vi "MasterRobotModeController.vi"() -> (1 "FMS Robot Mode":T1, 2 "Auto Reset":bool, 3 "Robot is Autonomous":bool)   [LabVIEW 2019]
doc: "This state controller manages the Robot Mode and whether or not the robot is running autonomously. The robot will continue running autonomously after Autonomous Mode ends, until the driver touches the joystick during TeleOperated Mode or until/unless the FORCE HUMAN CONTROL override is flipped on the FRC 4265 Dashboard."
uses:
  <vilib>/Rock Robotics/WPI/DriverStation/WPI_DriverStationRobotMode2.ctl
  refnums.vi
  GRNF_Joystick.vi
  dsdata.vi
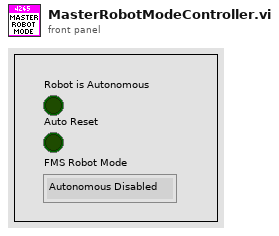
[diagram p1: front panel]
types:
  T1 = typedef "WPI_DriverStationRobotMode2.ctl" = enum16{"Autonomous Disabled", "Autonomous Enabled", "Teleop Disabled", "Teleop Enabled", "Disconnected", "Finish", "Test Disabled", "Test Enabled", "Emergency Stopped"}
  T2 = typedef "WPI_JoystickDevRef.ctl" = cluster{"Device":T3}
  T3 = typedef "WPI_JoystickDeviceEnum.ctl" = enum16{"USB 0", "USB 1", "USB 2", "USB 3", "USB 4", "USB 5"}
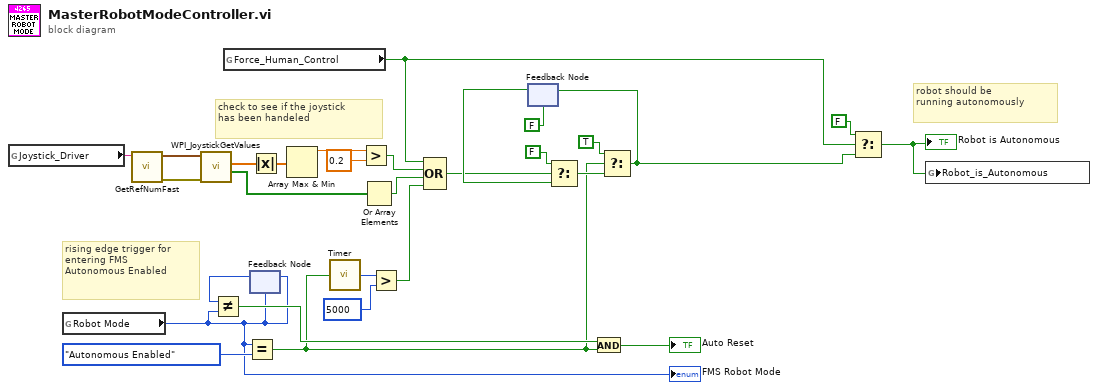
[diagram p0: block diagram]
diagram:
  # "rising edge trigger for\nentering FMS\nAutonomous Enabled"
  # "robot should be\nrunning autonomously"
  # "check to see if the joystick \nhas been handeled"
  n1 = global read "refnums.vi" "Joystick_Driver"() -> (w27:string)
  n2 = global read "dsdata.vi" "Robot Mode"() -> (w9:T1)
  "FMS Robot Mode" <- w9
  n3 = call-poly "GetRefNumFast.vi"("RefNum Name"=w27) -> ("Error"=w28:errorcluster, "Device Reference"=w29:T2)  [unwired: 5 in]
  n4 = call <vilib>:"WPI_JoystickGetValues.vi"("error in (no error)"=w28, "JoystickDevRef"=w29) -> ("Buttons"=w26:bool[], "Axes"=w25:dbl[])  [unwired: 5 in, 3 out]
  n5 = global read "dsdata.vi" "Force_Human_Control"() -> (w5:bool)
  n6 = Equal?(x=w9, y=WPI_DriverStationRobotMode2."Autonomous Enabled" ("Robot Mode")) -> (x = y?=w4:bool)
  n7 = feedback #1(w9) -> (w16:T1)
  n8 = Not Equal?(x=w16, y=w9) -> (x != y?=w15:bool)
  n9 = feedback-in #1(w9) -> ()
  n10 = Absolute Value(x=w25) -> (abs(x)=w24:dbl[])
  n11 = Array Max & Min(array=w24) -> (max value=w23:dbl)  [unwired: 3 out]
  n12 = call "Timer.vi"("Reset Timer"=w4) -> ("Time (ms)"=w3:u32)
  n13 = Greater?(x=w23, y=0.2) -> (0:w21:bool)
  n14 = Or Array Elements(Boolean array=w26) -> (logical OR=w20:bool)
  n15 = Greater?(x=w3, y=u32 5000) -> (0:w1:bool)
  n16 = Compound Arithmetic op=OR(w5, w21, w20, w1) -> (w10:bool)
  n17 = feedback #2(FALSE) -> (w11:bool)
  n18 = Select(t=FALSE, s=w10, f=w11) -> (s? t:f=w12:bool)
  n19 = And(x=w15, y=w4) -> (x .and. y?=→"Auto Reset":bool)
  n20 = Select(t=TRUE, s=w4, f=w12) -> (s? t:f=w7:bool)
  n21 = feedback-in #2(w7) -> ()
  n22 = Select(t=FALSE, s=w5, f=w7) -> (s? t:f=w6:bool)
  "Robot is Autonomous" <- w6
  n23 = global write "dsdata.vi" "Robot_is_Autonomous"(w6) -> ()
